vi "VI Scripting with Structures - Stacked Sequence Structure.vi"   [LabVIEW 2023]
doc: "This example contains sample code demonstrating common VI Scripting navigational tasks relating to Stacked Sequence Structures."
panel:
  # "Overview: Illustrates several Sequence properties and methods used for inspecting and modifying Stacked Sequence Structures with VI Scripting.\nInstructions:\nOpen the block diagram of this VI to see several examples of properties and methods related to Stacked Sequence Structures and VI Scripting.\n\nNote: Browse the diagram of this example to learn about VI Scripting concepts. This example is not meant to be run."
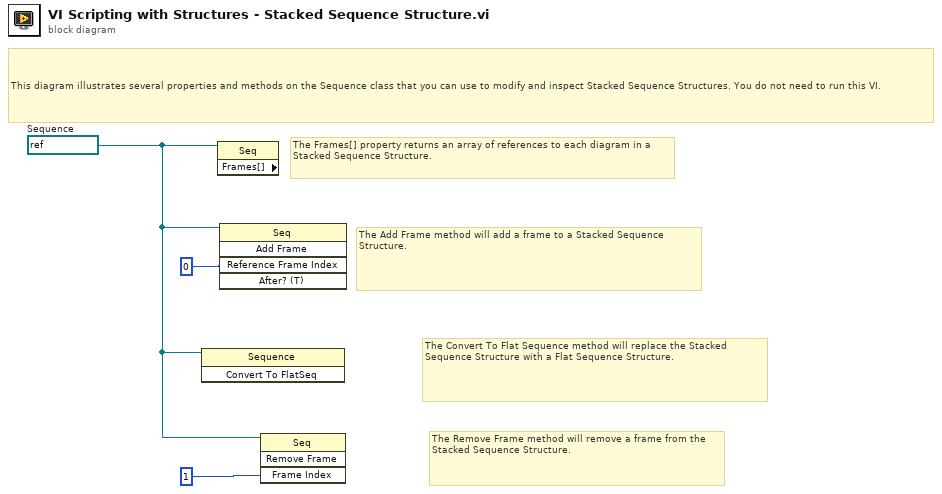
[diagram p0: block diagram]
diagram:
  w3 = refnum<vi> refnum  # Sequence
  # "The Convert To Flat Sequence method will replace the Stacked Sequence Structure with a Flat Sequence Structure."
  # "The Remove Frame method will remove a frame from the Stacked Sequence Structure."
  # "The Add Frame method will add a frame to a Stacked Sequence Structure."
  # "The Frames[] property returns an array of references to each diagram in a Stacked Sequence Structure."
  # "This diagram illustrates several properties and methods on the Sequence class that you can use to modify and inspect Stacked Sequence Structures. You do not need to run this VI."
  n1 = invoke class="Sequence" method="Convert To FlatSeq"(reference=w3) -> ()  [unwired: 2 in, 3 out]
  n2 = property class="Seq" props=["Frames[]"](reference=w3) -> ()  [unwired: 1 in, 3 out]
  n3 = invoke class="Seq" method="Add Frame"(reference=w3, "Reference Frame Index"=u32 0) -> ()  [unwired: 3 in, 5 out]
  n4 = invoke class="Seq" method="Remove Frame"(reference=w3, "Frame Index"=u32 1) -> ()  [unwired: 2 in, 4 out]
